vi "XY Graph Celsius vs Fahrenheit.vi"() -> ()   [LabVIEW 2019]
panel:
  out "Temperature comparisons":cluster{"X":dbl, "Y":dbl}[](graph)
  # "Challenge:\nCreate an xy graph that plots Celsius vs Fahrenheit temperatures."
  # "Try it: Run the program."
  # "You will probably need:\nXY graph, cluster, for loop, numeric functions"
  # "Open the block diagram to see a possible solution."
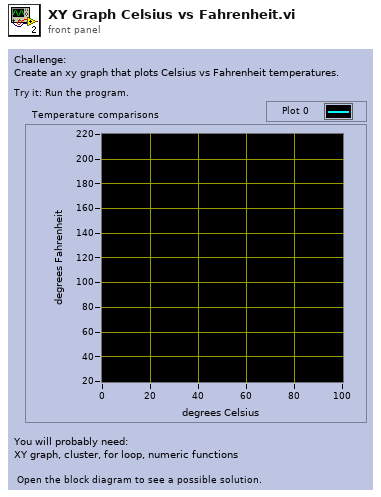
[diagram p1: front panel]
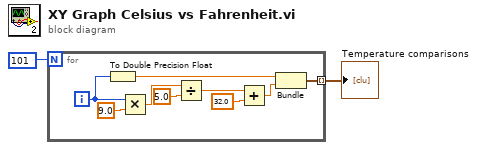
[diagram p0: block diagram]
diagram:
  n1 = for {
    N: 101 -> [_]
    tunnel: [w3] -> w1 mode=indexing
    i -> [w5]
    n2 = To Double Precision Float(number=w5) -> (double precision float=w4:dbl)
    n3 = Multiply(x=w5, y=9.0) -> (x*y=w8:dbl)
    n4 = Divide(x=w8, y=5.0) -> (x/y=w7:dbl)
    n5 = Add(x=w7, y=32.0) -> (x+y=w6:dbl)
    n6 = Bundle(w4, w6) -> (w3:cluster{dbl, dbl})  [unwired: 1 in]
  }
  "Temperature comparisons" <- w1
